vi "PM5000_factor_kW.vi"(1 "Data In":sgl[](array[numeric])) -> (0 "kW":sgl format="%#_4g")   [LabVIEW 2018]
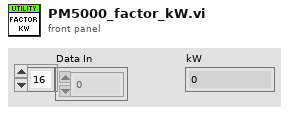
[diagram p1: front panel]
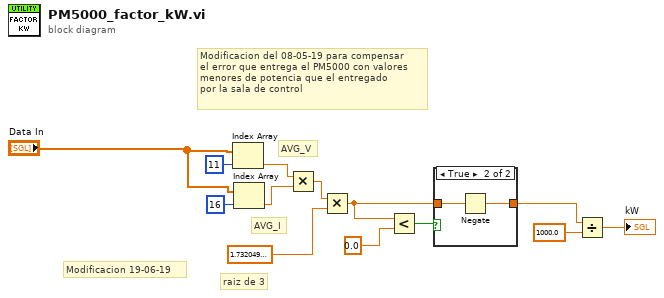
[diagram p0: block diagram]
diagram:
  # "Modificacion 19-06-19"
  # "Modificacion del 08-05-19 para compensar\nel error que entrega el PM5000 con valores\nmenores de potencia que el entregado \npor la sala de control"
  # "raiz de 3"
  # "AVG_I"
  # "AVG_V"
  n1 = Index Array(array="Data In", index=11) -> (element=w9:sgl)
  n2 = Index Array(array="Data In", index=16) -> (element=w10:sgl)
  n3 = Multiply(x=w9, y=w10) -> (x*y=w11:sgl)
  n4 = Multiply(x=w11, y=sgl 1.73205) -> (x*y=w13:sgl)
  n5 = Less?(x=w13, y=sgl 0.0) -> (x < y?=w4:bool)
  n6 = case shown="True" w4 {
    tunnel: w13 -> [w14 w16]
    tunnel: [w14 w15] -> w3
    frame False {
    }
    frame True {
      n7 = Negate(x=w16) -> (-x=w15:sgl)
    }
  }
  n8 = Divide(x=w3, y=sgl 1000.0) -> (x/y=→"kW":sgl)
